vi "Control System with Digital Twin - State Machine.vi"() -> ()   [LabVIEW 2021]
uses:
  <vilib>/Simulation/Scripting/Companion Diagram/SimConfigNode/SimParams.ctl
  <vilib>/Simulation/Scripting/Companion Diagram/SimConfigNode/_simSolvers.ctl
  <vilib>/Simulation/Implementation/Shared/SIMSCR Execution Mode.ctl
  <vilib>/Simulation/Param Hierarchy/Typedefs/SIMPH Param Control Actions.ctl
  <vilib>/Simulation/Implementation/Shared/NILVSim_ParamChanged.vi
  <vilib>/Simulation/Implementation/Shared/NILVSIM_BeginStep.vi
  <vilib>/Simulation/Implementation/Shared/NILVSim_Manager.vi
  <vilib>/Utility/error.llb/Clear Errors.vi
  <vilib>/Simulation/Implementation/Shared/NILVSim_FinalizeModel.vi
  <vilib>/Simulation/Implementation/Shared/SIM Unbundle Sim Info.vi
  <vilib>/Simulation/Implementation/Shared/NILVSim_Initialize.vi
  <vilib>/Simulation/Utility/Implementation/NILVSim Get Time and IsAcceptedStep.vi
  <vilib>/Simulation/Implementation/Shared/SIMSH Read Queue.vi
  <vilib>/Simulation/Implementation/Shared/NILVSim_GetModelError.vi
  <vilib>/Simulation/Implementation/Shared/SIM Bundle Sim Info.vi
  <vilib>/Simulation/Implementation/XNodeFramework/SimXNode/SimX.xnode
  Blackbox/Air Heater Black Box Model.vi
  <vilib>/Simulation/Scripting/Companion Diagram/SimConfigNode/SimDog.xnode
  SubVIs/Air Heater Model.vi
  <vilib>/Simulation/Implementation/Shared/NI_SIM_Implementation.lvlib
panel:
  out "Error [%]":dbl format="%.2g"
  out "Model [°C]":dbl format="%.2g"
  out "Control Chart":dbl(graph)=1.1724378087907898 caption="Controller Chart"
  in  "Stop Button":bool
  out "Measurement Chart":T1(graph)
  out "PV [°C]":dbl format="%.2g"
  out "MV [V]":dbl=1.0 format="%.2g"
  # "Process Value (PV)"
  # "Manipulated Value (MV)"
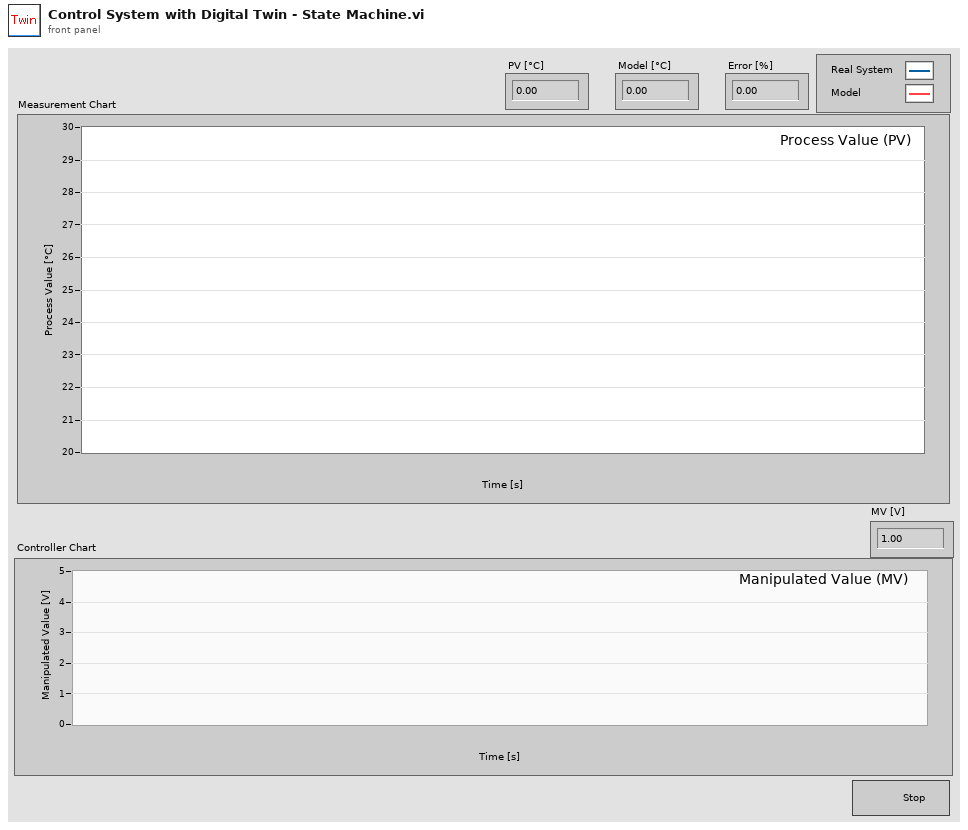
[diagram p1: front panel]
types:
  T1 = cluster{"Output Value [20-50degC]":dbl, "Tout [C]":dbl}
  T2 = cluster{"Output Value [20-50degC]":dbl, "Tout [C]":dbl}[]
  T3 = enum16{"Simulate to Completion", "Single Time-Step Simulation (Fixed Step Only)"}
  T4 = typedef "SIMSCR Execution Mode.ctl" = enum16{"Simulate to Completion", "Single Time-Step Simulation (Fixed Step Only)"}
  T5 = typedef "SIMPH Param Control Actions.ctl" = enum16{"get params", "set params"}
  T6 = cluster{"SIMSH Sim Time":dbl, "Linear Scaling with Points.vi 2":cluster{"Output":dbl}, "Select":cluster{"s? t:f":dbl}, "Summation 3":cluster{"Result":dbl}, "Square Root":cluster{"sqrt(x)":dbl}, "Gaussian White Noise PtByPt.vi":cluster{"Gaussian white noise":dbl}, "Integrator":cluster{"output":dbl}, "Multiplication":cluster{"Result":dbl}, "Summation":cluster{"Result":dbl}, "Multiplication 2":cluster{"Result":dbl}, "Transport Delay":cluster{"output":dbl}, "Summation 2":cluster{"Result":dbl}}
  T7 = typedef "SimParams.ctl" = cluster{"Initial Time (s)":dbl, "Final Time (s)":dbl, "Step Size (s)":dbl, "ODE Solver":T8, "Minimum Step Size (s)":dbl, "Maximum Step Size (s)":dbl, "Relative Tolerance":dbl, "Absolute Tolerance":dbl, "Software Timing":bool, "Initial Step Size (s)":dbl, "Automatic Fixed Step Size?":bool, "Automatic Discrete Step Size?":bool, "Discrete Step Size (s)":dbl, "Calculate using Time Step":bool, "Solver Wired?":bool, "Prev.Frm.Expected End":u64, "Prev.Frm.Actual End":u64, "Prev.Frm.Finished Late?":bool, "Prev.Iter.Expected End":u64, "Prev.Iter.Actual End":u64, "Prev.Iter.Finished Late?":bool, "Expected Iteration Start":u64, "Actual Iteration Start":u64, "Expected Frame Start":u64, "Actual Frame Start":u64, "Source Name":string, "Name":string, "Period":i64, "Deadline":i64, "Offset":i64, "Start":i64, "Priority":i32, "Timeout":i32, "Processor":i32, "Mode":enum32{"No Change", "Process missed periods, maintain original phase", "Discard missed periods, maintain original phase", "Process missed periods, ignore original phase", "Discard missed periods, ignore original phase"}, "Wakeup reason":enum32{"Normal", "Aborted", "Asynchronous wakeup", "Timing source error", "Timed loop error", "Timeout"}, "Error":errorcluster, "Source Type":string, "Secondary Source Type":string, "Global End Time":u64, "Global Start Time":u64, "Full Solver Reset":bool, "Execution Mode":T4, "Nan/Inf Check":bool, "Custom Solver Library":string, "Solver Is Variable":bool, "custom solver name":string, "Signal Collection Decimation":u32}
  T8 = typedef "_simSolvers.ctl" = enum16{"Runge-Kutta 1 (Euler)", "Runge-Kutta 2", "Runge-Kutta 3", "Runge-Kutta 4", "Runge-Kutta 23 (variable)", "Runge-Kutta 45 (variable)", "BDF (variable)", "Adams-Moulton (variable)", "Rosenbrock (variable)", "Discrete States Only", "SDIRK 4 (variable)", "Radau 5 (variable)", "Radau 9 (variable)", "Radau 13 (variable)", "Radau [Variable Order] (variable)", "Gear's Method (variable)", "Linearizer", "State Query", "Trim Eval", "Custom Solver"}
  T9 = cluster{"SIMSH Sim Time":dbl, "lower limit":dbl, "Integrator":cluster{"output":dbl}, "Multiplication":cluster{"Result":dbl}, "Summation":cluster{"Result":dbl}, "Multiplication 2":cluster{"Result":dbl}, "Transport Delay":cluster{"output":dbl}, "Summation 2":cluster{"Result":dbl}}
  T10 = cluster{"T_init [C]":dbl, "T [s]":dbl, "K [C/V]":dbl, "T_delay [s]":dbl, "T_env [C]":dbl}
  T11 = enum16{"LabVIEW PID", "Fuji Blackbox", "Real Fuji PID"}
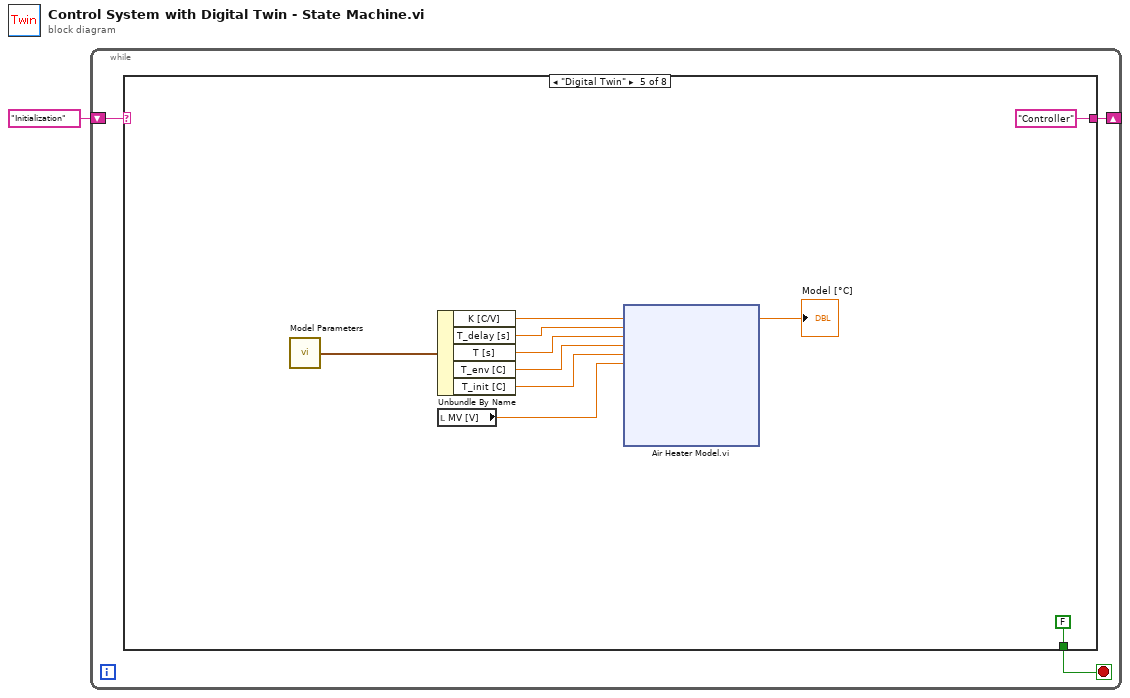
[diagram p0: block diagram]
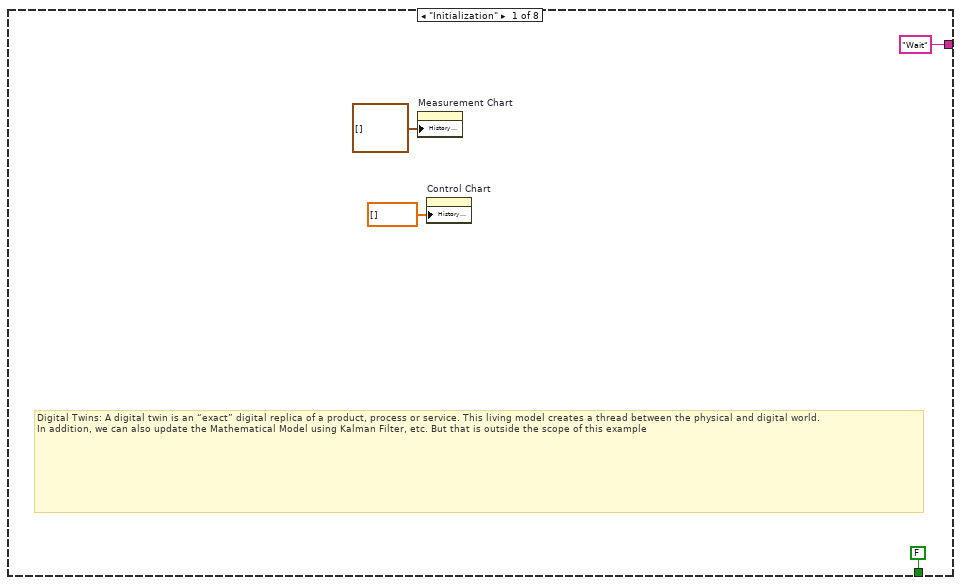
[diagram p2: hidden frame]
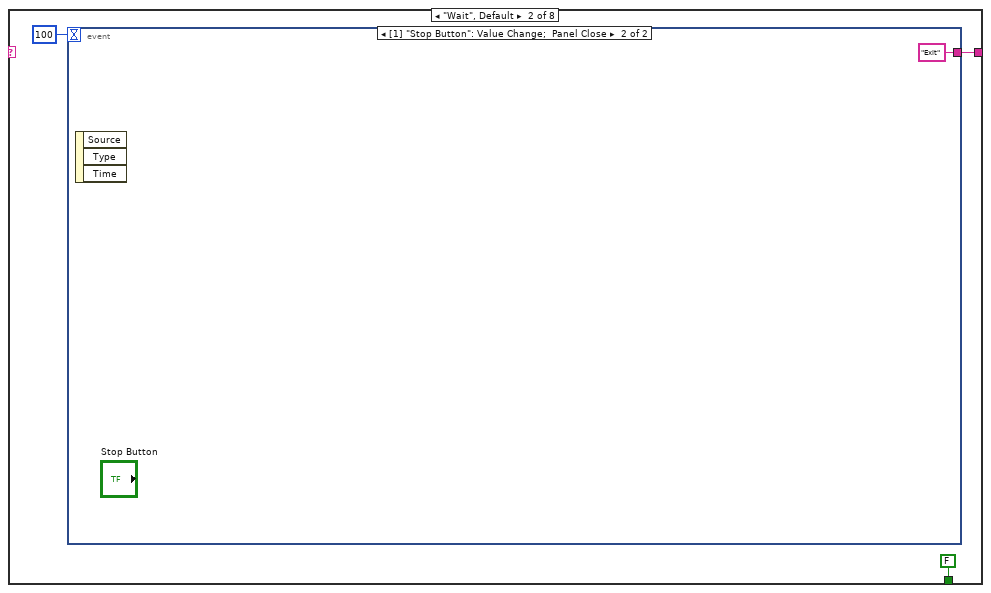
[diagram p3: hidden frame]
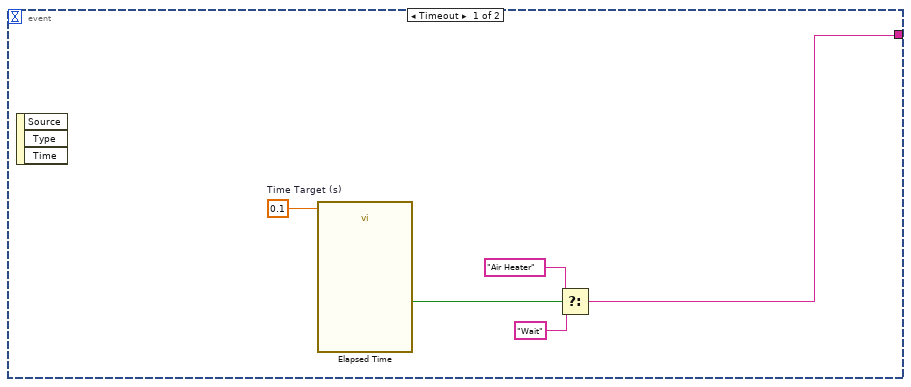
[diagram p4: hidden frame]
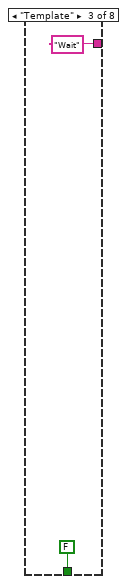
[diagram p5: hidden frame]
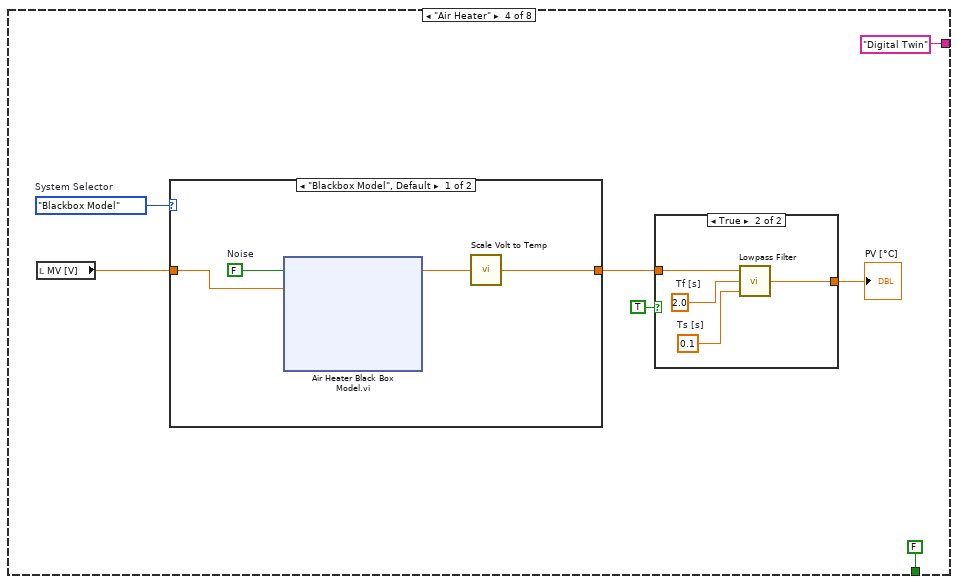
[diagram p6: hidden frame]
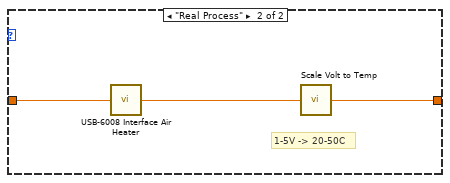
[diagram p8: hidden frame]
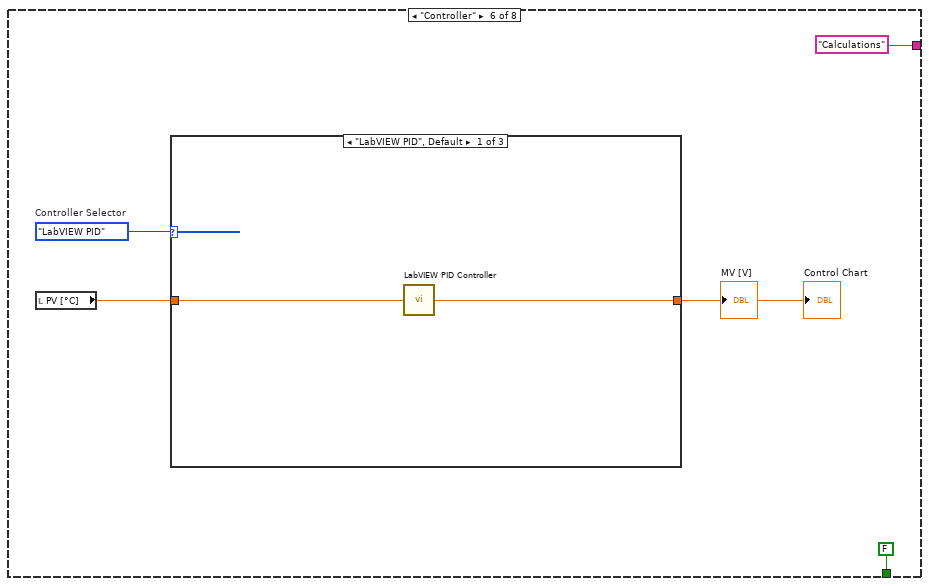
[diagram p9: hidden frame]
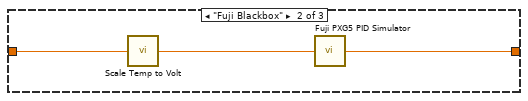
[diagram p10: hidden frame]
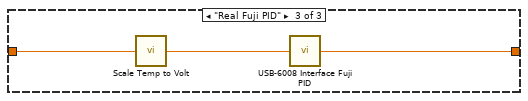
[diagram p11: hidden frame]
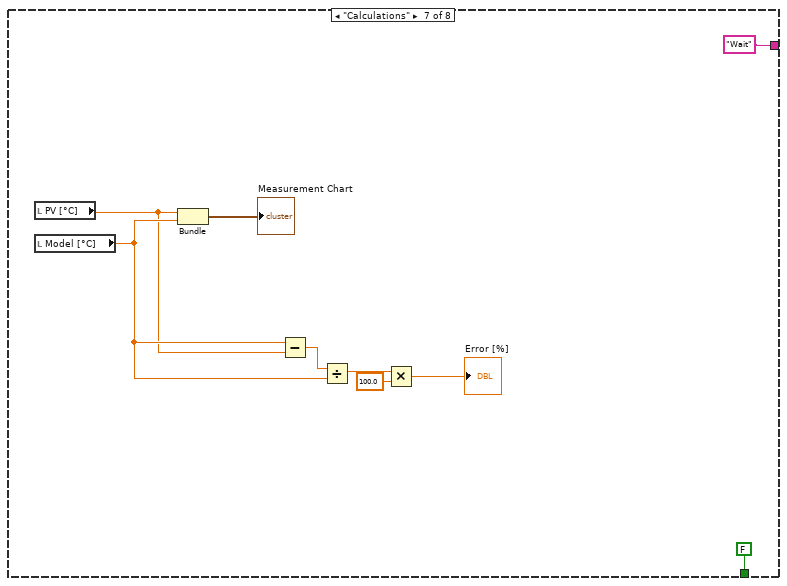
[diagram p12: hidden frame]
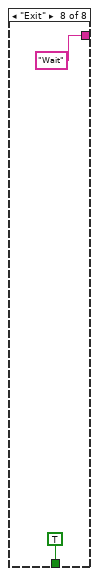
[diagram p13: hidden frame]
diagram:
  n1 = while {
    shift-right: [w3] -> _
    shift-left: "Initialization" -> [w4]
    stop <- w2 stop-if-true
    n2 = case shown="\"Digital Twin\"" w4 {
      tunnel: ["Wait" w9 "Wait" "Digital Twin" "Controller" "Calculations" "Wait" "Wait"] -> w3
      tunnel: [FALSE FALSE FALSE FALSE FALSE FALSE FALSE TRUE] -> w2
      frame "Initialization" {
        # "Digital Twins: A digital twin is an “exact” digital replica of a product, process or service. This living model creates a thread between the physical and digital world.\nIn addition, we can also update the Mathematical Model using Kalman Filter, etc. But that is outside the scope of this example"
        n3 = property on="Measurement Chart" class="WFChart (strict)"("History Data"=T2 []) -> ()  [unwired: 2 in, 2 out]
        n4 = property on="Control Chart" class="WFChart (strict)"("History Data"=dbl[] []) -> ()  [unwired: 2 in, 2 out]
      }
      frame "Wait", Default {
        n5 = event shown="[1] \"Stop Button\": Value Change;  Panel Close" {
          selector: _ -> [_ _]
          dyn-events: _ -> [_ _]
          timeout: 100 ("ms") -> [_ _]
          tunnel: [w12 "Exit"] -> w9
          event Timeout {
            w13 = 0.1  # Time Target (s)
            n6 = event-data() -> ()  [unwired: 1 in, 3 out]
            n7 = call "Elapsed Time"("Time Target (s)"=w13) -> ("Time has Elapsed"=w16:bool)  [unwired: 11 in, 7 out]
            n8 = Select(t="Air Heater", s=w16, f="Wait") -> (s? t:f=w12:string)
          }
          event "Stop Button": Value Change; Panel Close {
            n9 = event-data() -> ()  [unwired: 1 in, 3 out]
          }
        }
      }
      frame "Template" {
      }
      frame "Air Heater" {
        w24 = enum16{"Blackbox Model", "Real Process"}."Blackbox Model"  # System Selector
        n10 = local read "MV [V]"() -> (w23:dbl)
        n11 = case shown="\"Blackbox Model\", Default" w24 {
          tunnel: [w34 w292] -> w22
          tunnel: w23 -> [w33 w291]
          frame "Blackbox Model", Default {
            w32 = FALSE  # Noise
            n12 = xnode "Air Heater Black Box Model.vi"("Noise"=w32, "Control Signal [0-5V]"=w33) -> ("Tout [1-5V]"=w35:dbl)  [unwired: 3 in, 1 out]
            n13 = call "Scale Volt to Temp.vi"("Input Value [1-5V]"=w35) -> ("Output Value [20-50degC]"=w34:dbl)
          }
          frame "Real Process" {
            # "1-5V -> 20-50C"
            n14 = call "USB-6008 Interface Air Heater.vi"("Control Signal [0-5V]"=w291) -> ("Process Value [1-5V]"=w293:dbl)
            n15 = call "Scale Volt to Temp.vi"("Input Value [1-5V]"=w293) -> ("Output Value [20-50degC]"=w292:dbl)
          }
        }
        n16 = case shown="True" TRUE {
          tunnel: w22 -> [w27 w31]
          tunnel: [w27 w30] -> w21
          frame False {
          }
          frame True {
            w28 = 2.0  # Tf [s]
            w29 = 0.1  # Ts [s]
            n17 = call "Lowpass Filter.vi"("Ts [s]"=w29, "Tf [s]"=w28, "Filter Input"=w31) -> ("Filter Output"=w30:dbl)
          }
        }
        "PV [°C]" <- w21
      }
      frame "Digital Twin" {
        n18 = call "Model Parameters.vi"() -> ("Model Parameters Out"=w294:T10)  [unwired: 1 in]
        n19 = Unbundle By Name(w294) -> ("K [C/V]"=w296:dbl, "T_delay [s]"=w297:dbl, "T [s]"=w298:dbl, "T_env [C]"=w299:dbl, "T_init [C]"=w300:dbl)
        n20 = local read "MV [V]"() -> (w295:dbl)
        n21 = xnode "Air Heater Model.vi"("K [C/V]"=w296, "T_delay [s]"=w297, "T [s]"=w298, "T_env [C]"=w299, "T_init [C]"=w300, "u [V]"=w295) -> ("Tout [C]"=→"Model [°C]":dbl)  [unwired: 2 in, 10 out]
      }
      frame "Controller" {
        w577 = T11."LabVIEW PID"  # Controller Selector
        n22 = local read "PV [°C]"() -> (w576:dbl)
        n23 = case shown="\"LabVIEW PID\", Default" w577 {
          tunnel: [w581 w585 w587] -> w578
          tunnel: w576 -> [w582 w583 w586]
          frame "LabVIEW PID", Default {
            n24 = call "LabVIEW PID Controller.vi"("PV [°C]"=w582) -> ("MV [0-5V]"=w581:dbl)
          }
          frame "Fuji Blackbox" {
            n25 = call "Scale Temp to Volt.vi"("Input Value [20-50degC]"=w583) -> ("Output Value [1-5V]"=w584:dbl)
            n26 = call "Fuji PXG5 PID Simulator.vi"("Input (1-5V)"=w584) -> ("Output (0-5V)"=w585:dbl)
          }
          frame "Real Fuji PID" {
            n27 = call "Scale Temp to Volt.vi"("Input Value [20-50degC]"=w586) -> ("Output Value [1-5V]"=w588:dbl)
            n28 = call "USB-6008 Interface Fuji PID.vi"("Process Value  [1-5V]"=w588) -> ("Control Value [0-5V]"=w587:dbl)
          }
        }
        "MV [V]" <- w578
        "Control Chart" <- w578
      }
      frame "Calculations" {
        n29 = local read "PV [°C]"() -> (w589:dbl)
        n30 = local read "Model [°C]"() -> (w590:dbl)
        n31 = Bundle("PV [°C]"=w589, "Model [°C]"=w590) -> (→"Measurement Chart":cluster{"PV [°C]":dbl, "Model [°C]":dbl})  [unwired: 1 in]
        n32 = Subtract(x=w590, y=w589) -> (x-y=w593:dbl)
        n33 = Divide(x=w593, y=w590) -> (x/y=w594:dbl)
        n34 = Multiply(x=w594, y=100.0) -> (x*y=→"Error [%]":dbl)
      }
      frame "Exit" {
      }
    }
  }
